vi "Host Help Text.vi"() -> (3 "Help Text":string)   [LabVIEW 2019]
panel:
  in  "version":string="3.0"
  in  "cmds":cluster{"cmd":string, "desc":string}[](array[cluster])=[{"cmd"="?", "desc"="Short Status"}, {"cmd"="+", "desc"="Full Status"}, {"cmd"="ST", "desc"="Stop all motion"}, {"cmd"="CL", "desc"="Close Main Door"}, {"cmd"="OP", "desc"="Open Main Door"}, {"cmd"="UP", "desc"="Close (rise) Dropout Door"}, {"cmd"="DN", "desc"="Open (lower) Dropout Door"}, {"cmd"="SO", "desc"="Synchronized Open (Both doors open together)"}, {"cmd"="SC", "desc"="Synchronized Close (Both doors close together)"}, {"cmd"="AO", "desc"="Auto shutdown ON"}, {"cmd"="AF", "desc"="Auto shutdown OFF"}, {"cmd"="CO", "desc"="Cloud Sensor ON"}, {"cmd"="CF", "desc"="Cloud Sensor OFF"}, {"cmd"="CN", "desc"="Rotate to encoder center position"}, {"cmd"="HM", "desc"="Rotate to home position"}, {"cmd"="d MV", "desc"="Move to Azimuth (d=degrees,0.0<=d<360)"}, {"cmd"="d TOL", "desc"="Tolerance (d=degrees,0.0<=d<3)"}, {"cmd"="d HZ", "desc"="Define home position (d=degrees,0.0<=d<360)"}, {"cmd"="d HS", "desc"="High speed threshold (d=degrees,0.0<=d<10)"}, {"cmd"="d LM", "desc"="Encoder counts for 360 degrees"}, {"cmd"="t WT", "desc"="Watchdog Timer (t=seconds,600 typical)"}, {"cmd"="t RD", "desc"="Set reverse direction motion delay (t=seconds,0<=t<6)"}, {"cmd"="t AT", "desc"="Set Azimuth motion timeout (t=seconds,120<=t<600)"}, {"cmd"="t RS", "desc"="Set Rain / Cloud activate delay (t=seconds,1<=t<10)"}, {"cmd"="AEP", "desc"="AZ Encoder Count Positive"}, {"cmd"="AEN", "desc"="AZ Encoder Count Negative"}, {"cmd"="CFS", "desc"="Save current configuration"}, {"cmd"="CFR", "desc"="Recall last saved configuration"}, {"cmd"="AWO", "desc"="Private control link ON (WIFI-6 antenna)"}, {"cmd"="AWF", "desc"="Private control link OFF (WIFI-6 antenna)"}, {"cmd"="AWA", "desc"="Private remote antenna is alive? (WIFI-6 antenna)"}, {"cmd"="AWC", "desc"="Private local antenna connections (WIFI-6 antenna)"}, {"cmd"="AWR", "desc"="Private local antenna reboot command (WIFI-6 antenna)"}, {"cmd"="HELP", "desc"="Display this list of available commands"}]
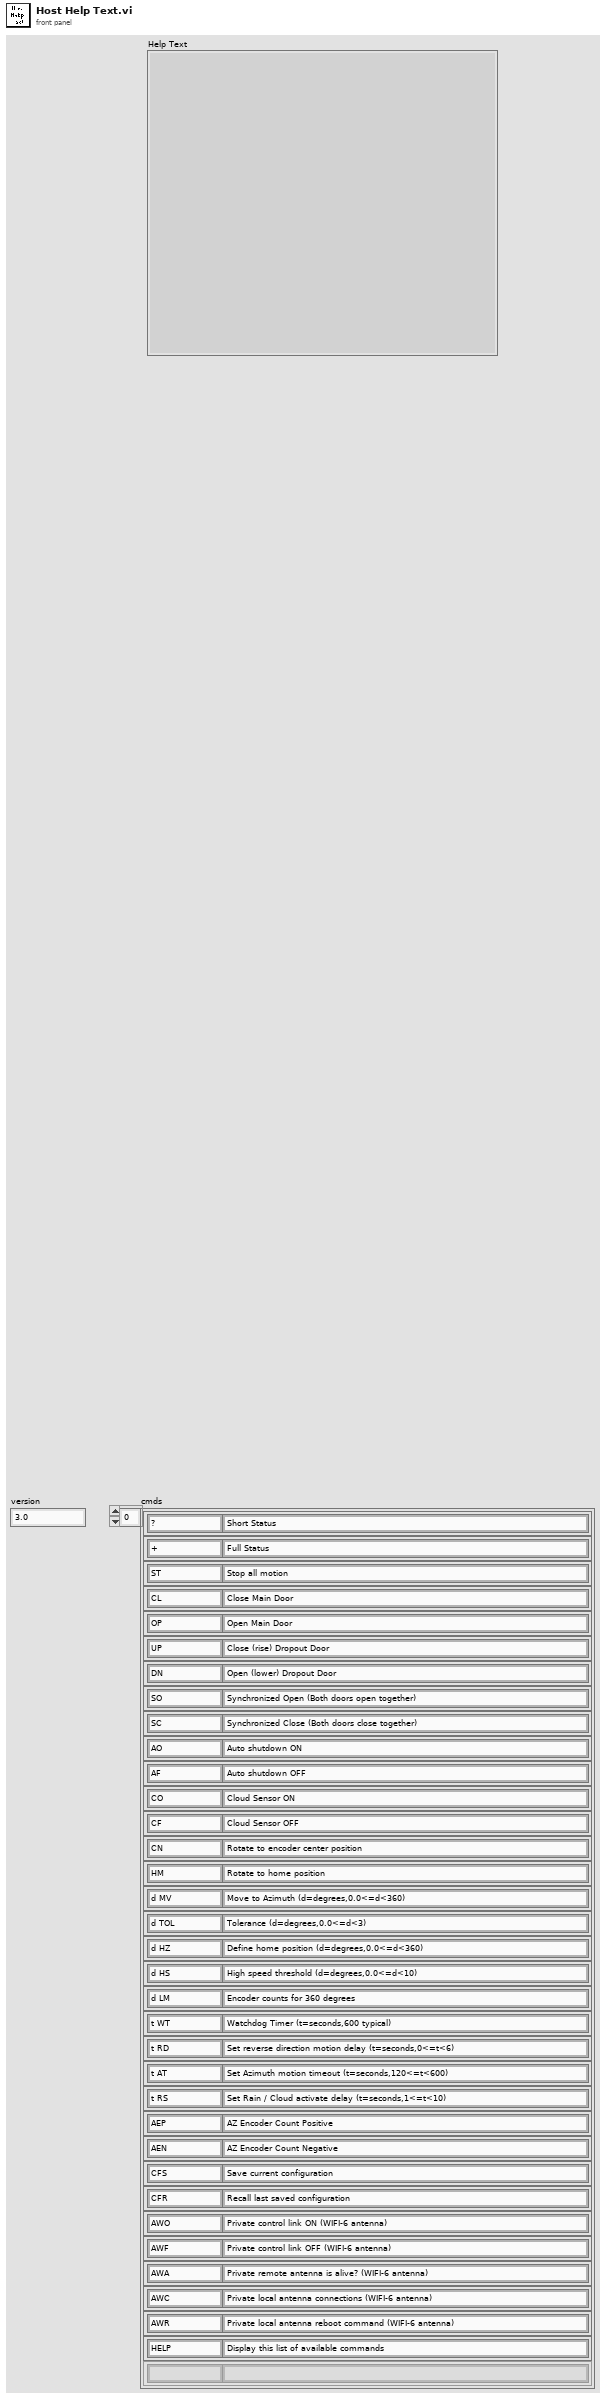
[diagram p1: front panel]
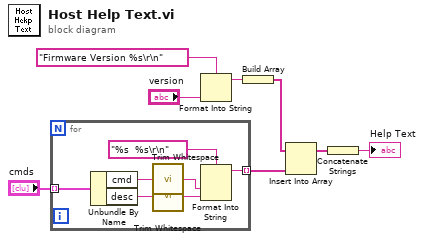
[diagram p0: block diagram]
diagram:
  n1 = for {
    tunnel: "cmds" -> [w15] mode=indexing
    tunnel: [w13] -> w8 mode=indexing
    n2 = Unbundle By Name(w15) -> ("cmd"=w12:string, "desc"=w10:string)
    n3 = call <vilib>:"Trim Whitespace.vi"("string"=w12) -> ("trimmed string"=w11:string)  [unwired: 1 in]
    n4 = call <vilib>:"Trim Whitespace.vi"("string"=w10) -> ("trimmed string"=w9:string)  [unwired: 1 in]
    n5 = Format Into String(format string="%s  %s\r\n", w11, w9) -> (resulting string=w13:string)  [unwired: 2 in, 1 out]
  }
  n6 = Format Into String(format string="Firmware Version %s\r\n", "version") -> (resulting string=w5:string)  [unwired: 2 in, 1 out]
  n7 = Build Array(w5) -> (w4:string[])
  n8 = Insert Into Array(array=w4, new element=w8) -> (w3:string[])  [unwired: 1 in]
  n9 = Concatenate Strings(w3) -> (→"Help Text":string)
